vi "Find Table Cell from Coordinate.vi"(8 "error in (no error)":errorcluster, 10 "Coords":T1, 11 "MCLB Refs":refnum<vi>) -> (0 "error out":errorcluster, 1 "Found?":bool, 2 "Column":u32, 3 "Row":u32)   [LabVIEW 2020]
uses:
  <vilib>/Utility/miscctls.llb/LVPoint32TypeDef.ctl
  <vilib>/Utility/miscctls.llb/LVRowAndColumnUnsignedTypeDef.ctl
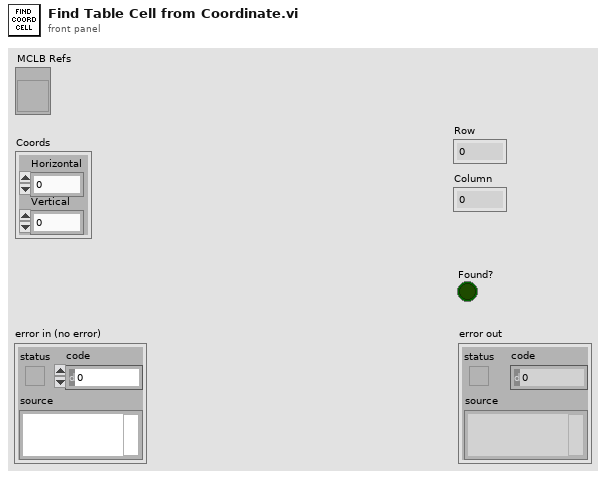
[diagram p1: front panel]
types:
  T1 = typedef "LVPoint32TypeDef.ctl" = cluster{"Horizontal":i32, "Vertical":i32}
  T2 = typedef "LVRowAndColumnUnsignedTypeDef.ctl" = cluster{"Row":u32, "Column":u32}
  T3 = typedef "LVBoundsTypeDef.ctl" = cluster{"Width":u32, "Height":u32}
  T4 = typedef "LVPositionTypeDef.ctl" = cluster{"Left":i32, "Top":i32}
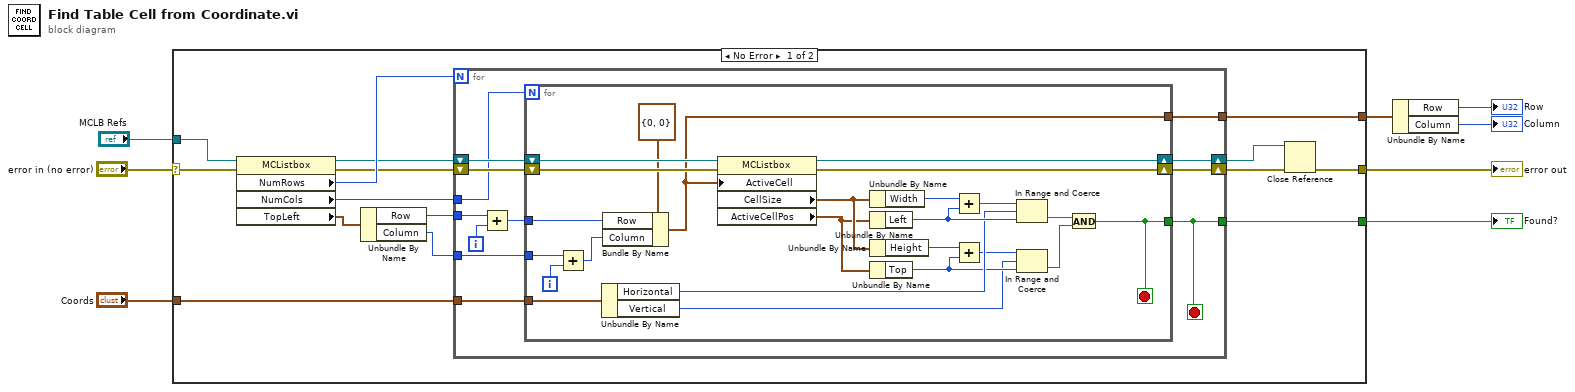
[diagram p0: block diagram]
diagram:
  n1 = case shown="No Error" "error in (no error)" {
    selector: "error in (no error)" -> [w23 w60]
    tunnel: [w11 w60] -> w7
    tunnel: "Coords" -> [w17 _]
    tunnel: [w16 _] -> w5
    tunnel: [w15 _] -> w3
    tunnel: "MCLB Refs" -> [w13 _]
    frame No Error {
      n2 = property class="MCListbox"(reference=w13, error in=w23) -> (reference out=w20:refnum<vi>, error out=w19:errorcluster, "NumRows"=w22:u32, "NumCols"=w18:u32, "TopLeft"=w14:T2)
      n3 = Unbundle By Name(w14) -> ("Row"=w21:u32, "Column"=w9:u32)
      n4 = for {
        N: w22 -> [_]
        tunnel: w21 -> [w35]
        shift-right: [w32] -> w10
        shift-left: w20 -> [w33]
        shift-right: [w30] -> w12
        shift-left: w19 -> [w31]
        tunnel: w18 -> [w29]
        tunnel: w17 -> [w27]
        tunnel: [w26] -> w16
        tunnel: [w25] -> w15
        tunnel: w9 -> [w24]
        i -> [w34]
        stop <- w26 stop-if-true
        n5 = Add(x=w35, y=w34) -> (x+y=w28:u32)
        n6 = for {
          N: w29 -> [_]
          shift-right: [w58] -> w32
          shift-left: w33 -> [w59]
          shift-right: [w56] -> w30
          shift-left: w31 -> [w57]
          tunnel: w28 -> [w54]
          tunnel: w27 -> [w50]
          tunnel: [w40] -> w26
          tunnel: [w39] -> w25
          tunnel: w24 -> [w37]
          i -> [w38]
          stop <- w40 stop-if-true
          n7 = Add(x=w37, y=w38) -> (x+y=w36:u32)
          n8 = Unbundle By Name(w50) -> ("Horizontal"=w49:i32, "Vertical"=w43:i32)
          n9 = Bundle By Name(cluster=T2 {"Row"=0, "Column"=0} ("Index Values"), "Row"=w54, "Column"=w36) -> (w39:T2)
          n10 = property class="MCListbox"(reference=w59, error in=w57, "ActiveCell"=w39) -> (reference out=w58:refnum<vi>, error out=w56:errorcluster, "CellSize"=w48:T3, "ActiveCellPos"=w47:T4)
          n11 = Unbundle By Name(w48) -> ("Width"=w53:u32)
          n12 = Unbundle By Name(w47) -> ("Left"=w52:i32)
          n13 = Unbundle By Name(w48) -> ("Height"=w46:u32)
          n14 = Unbundle By Name(w47) -> ("Top"=w44:i32)
          n15 = Add(x=w53, y=w52) -> (x+y=w51:u32)
          n16 = Add(x=w46, y=w44) -> (x+y=w45:u32)
          n17 = In Range and Coerce(upper limit=w51, x=w49, lower limit=w52) -> (In Range?=w42:bool)  [unwired: 1 out]
          n18 = In Range and Coerce(upper limit=w45, x=w43, lower limit=w44) -> (In Range?=w41:bool)  [unwired: 1 out]
          n19 = And(x=w42, y=w41) -> (x .and. y?=w40:bool)
        }
      }
      n20 = Close Reference(reference=w10, error in (no error)=w12) -> (error out=w11:errorcluster)
    }
    frame Error {
    }
  }
  "error out" <- w7
  "Found?" <- w5
  n21 = Unbundle By Name(w3) -> ("Row"=→"Row":u32, "Column"=→"Column":u32)
